vi "extract ending.vi"(10 "length":dbl=0.5 format="%#_13g", 11 "all rows":dbl[](array[numeric])) -> (3 "Array":dbl[](array[numeric]))   [LabVIEW 2015]
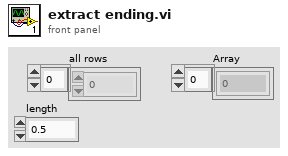
[diagram p1: front panel]
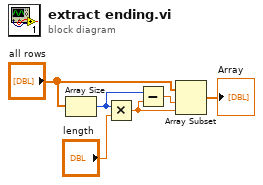
[diagram p0: block diagram]
diagram:
  n1 = Array Size(array="all rows") -> (size(s)=w4:i32)
  n2 = Multiply(x=w4, y="length") -> (x*y=w3:dbl)
  n3 = Subtract(x=w4, y=w3) -> (x-y=w5:dbl)
  n4 = Array Subset(array="all rows", index=w5, length=w3) -> (→"Array":dbl[])
